vi "integrator.vi"(1 "In":i16) -> (0 "Out":i16)   [LabVIEW 2010, in "Wall Follower.lvrbt"]
uses:
  Wall Follower.lvrbt
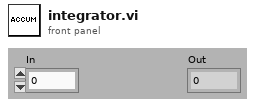
[diagram p1: front panel]
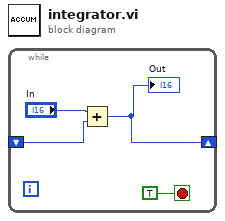
[diagram p0: block diagram]
diagram:
  n1 = while {
    shift-right: [w2] -> _
    shift-left: _ -> [w1]
    stop <- TRUE stop-if-true
    n2 = Add(x="In", y=w1) -> (x+y=w2:i16)
    "Out" <- w2
  }
